vi "Get Inverted Vertex.vi"(7 "Axis":enum16{"X-Axis", "Y-Axis", "Z-Axis"}(ring), 8 "Inverted?":T1, 9 "Range In":cluster{"Max":sgl, "Min":sgl}, 10 "Normal Array In":sgl[](array[numeric]), 11 "Vertex Array In":sgl[](array[numeric])) -> (2 "Normal Array Out":sgl[](array[numeric]), 3 "Vertex Array Out":sgl[](array[numeric]))   [LabVIEW 2017, in "3D Plot.lvclass"]
uses:
  <vilib>/Math Plots/3D Math Plots/3D Plot/3D Plot/3D Plot.lvclass
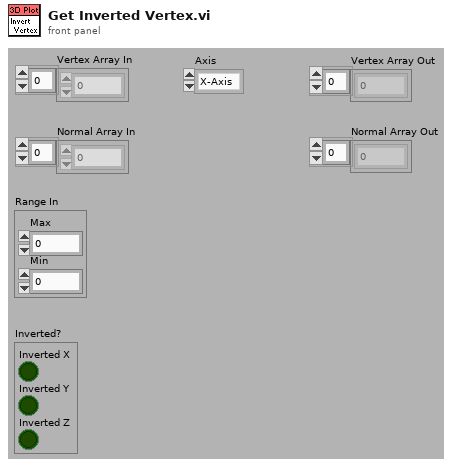
[diagram p1: front panel]
types:
  T1 = cluster{"Inverted X":bool, "Inverted Y":bool, "Inverted Z":bool}
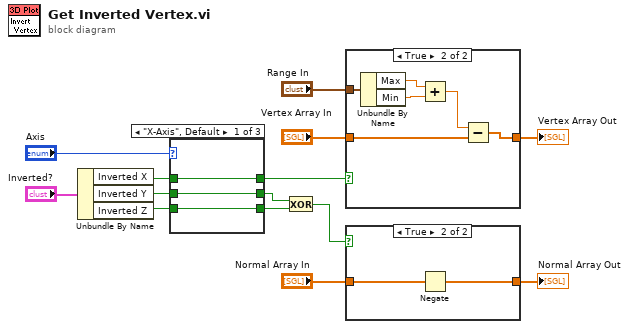
[diagram p0: block diagram]
diagram:
  n1 = Unbundle By Name("Inverted?") -> ("Inverted X"=w7:bool, "Inverted Y"=w6:bool, "Inverted Z"=w5:bool)
  n2 = case shown="\"X-Axis\", Default" "Axis" {
    tunnel: w7 -> [w17 w19 w22]
    tunnel: [w17 w20 w23] -> w1
    tunnel: w6 -> [w16 w20 w21]
    tunnel: w5 -> [w15 w18 w23]
    tunnel: [w16 w19 w22] -> w4
    tunnel: [w15 w18 w21] -> w3
    frame "X-Axis", Default {
    }
    frame "Y-Axis" {
    }
    frame "Z-Axis" {
    }
  }
  n3 = Exclusive Or(1:w3, 2:w4) -> (0:w2:bool)
  n4 = case shown="True" w1 {
    tunnel: "Vertex Array In" -> [w24 w25]
    tunnel: [w24 w26] -> w12
    tunnel: "Range In" -> [_ w30]
    frame False {
    }
    frame True {
      n5 = Unbundle By Name(w30) -> ("Max"=w29:sgl, "Min"=w28:sgl)
      n6 = Add(x=w29, y=w28) -> (x+y=w27:sgl)
      n7 = Subtract(x=w27, y=w25) -> (x-y=w26:sgl[])
    }
  }
  "Vertex Array Out" <- w12
  n8 = case shown="True" w2 {
    tunnel: "Normal Array In" -> [w31 w33]
    tunnel: [w31 w32] -> w10
    frame False {
    }
    frame True {
      n9 = Negate(x=w33) -> (-x=w32:sgl[])
    }
  }
  "Normal Array Out" <- w10
